vi "Submit Goal.vi"(8 "error in (no error)":errorcluster, 10 "Goal":dbl format="%#_13g", 11 "Generic Optimizer in":refnum<class "Generic Optimizer.lvclass">) -> (0 "error out":errorcluster, 3 "Generic Optimizer out":refnum<class "Generic Optimizer.lvclass">)   [LabVIEW 2020, in "RxnRover.lvlib" / "Generic Optimizer.lvclass"]
uses:
  Generic Optimizer.lvclass
  Generic Optimizer.lvclass/Generic Optimizer.ctl
  <userlib>/RxnRover/DynamicReentrant/Dynamic Reentrant.lvlib
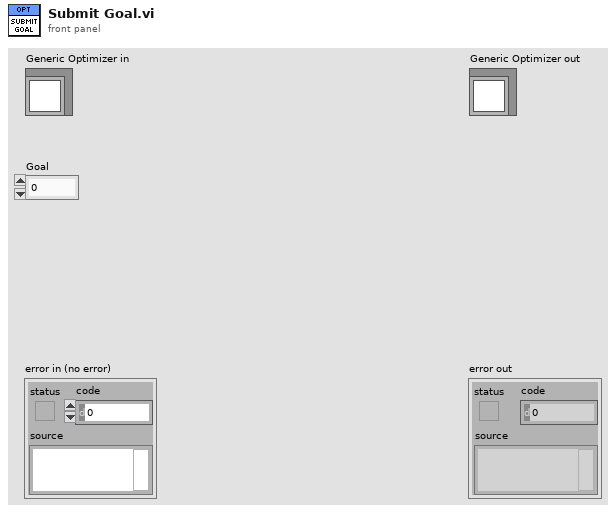
[diagram p1: front panel]
types:
  T1 = typedef "Dynamic Reentrant.lvlib/Message.ctl" = cluster{"Source":string, "Destination":string, "Time Stamp":timestamp, "Command":string, "Data":variant}
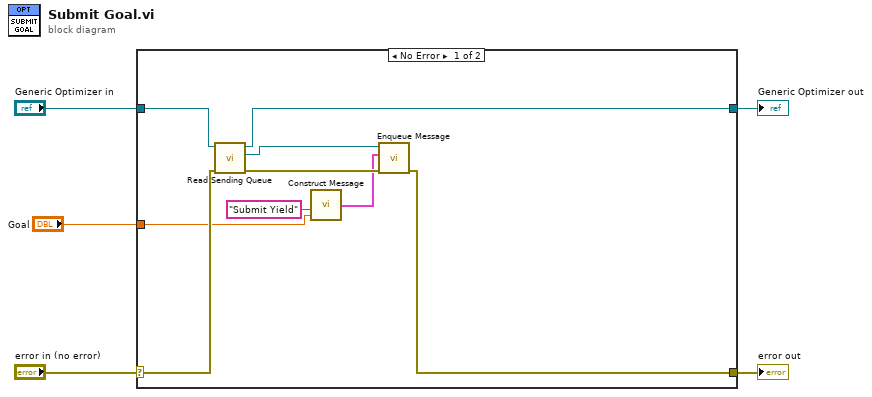
[diagram p0: block diagram]
diagram:
  n1 = case shown="No Error" "error in (no error)" {
    selector: "error in (no error)" -> [w14 w16]
    tunnel: [w6 w16] -> w4
    tunnel: [w12 w15] -> w2
    tunnel: "Generic Optimizer in" -> [w13 w15]
    tunnel: "Goal" -> [w8 _]
    frame No Error {
      n2 = call-dynamic "Read Sending Queue.vi"("error in (no error)"=w14, "Generic Controller in"=w13) -> ("error out"=w11:errorcluster, "Sending Queue"=w10:refnum<queue>, "Generic Controller out"=w12:refnum<class "Generic Optimizer.lvclass">)  [unwired: 7 in]
      n3 = call <userlib>:"Construct Message.vi"("Data"=w8, "Command"="Submit Yield") -> ("Message Cluster"=w7:T1)  [unwired: 4 in]
      n4 = call <userlib>:"Enqueue Message.vi"("error in (no error)"=w11, "Message"=w7, "Listening Queue"=w10) -> ("error out"=w6:errorcluster)  [unwired: 7 in, 1 out]
    }
    frame Error {
    }
  }
  "error out" <- w4
  "Generic Optimizer out" <- w2
